vi "Plot Update Cursor 3D Surface.vi"(8 "Cursor XYZ":T1, 11 "3D Surface":refnum<vi>) -> ()   [LabVIEW 2016]
uses:
  <vilib>/Math Plots/3D Math Plots/3D Surface/3D Surface XCtrl/3D Surface.xctl
  <vilib>/addons/Software Calibration Management/xSCM/Controls/TLU2D.ctl
  <vilib>/Math Plots/3D Math Plots/3D Plot/3D Plot/Typedef/Sprite Type.ctl
  <vilib>/Math Plots/3D Math Plots/3D Plot/3D Plot/3D Plot.lvclass
  <vilib>/addons/Software Calibration Management/xSCM/SCM-API.lvlib
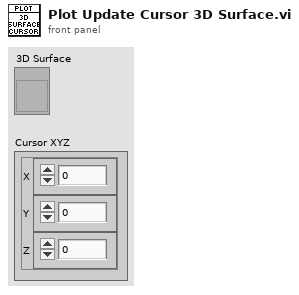
[diagram p1: front panel]
types:
  T1 = typedef "SCM-API.lvlib/TLU2D.ctl" = cluster{"X":sgl, "Y":sgl, "Z":sgl}
  T2 = typedef "3D Plot.lvclass/Sprite Type.ctl" = enum16{"None", "Empty Square", "Solid Square", "Empty Diamond", "Solid Diamond", "Empty Circle", "Solid Circle", "Asterisk", "Bold X", "Wireframe Sphere", "Solid Sphere", "Wireframe Cube", "Solid Cube"}
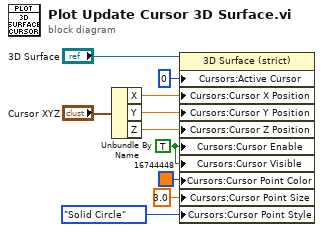
[diagram p0: block diagram]
diagram:
  w4 = TRUE ("Cursors:General:Cursor Enable")
  n1 = Unbundle By Name("Cursor XYZ") -> ("X"=w8:sgl, "Y"=w7:sgl, "Z"=w6:sgl)
  n2 = property class="3D Surface (strict)"(reference="3D Surface", "Cursors:Active Cursor"=0, "Cursors:Cursor X Position"=w8, "Cursors:Cursor Y Position"=w7, "Cursors:Cursor Z Position"=w6, "Cursors:Cursor Enable"=w4, "Cursors:Cursor Visible"=w4, "Cursors:Cursor Point Color"=u32 16744448 ("Cursors:Point:Cursor Point Color"), "Cursors:Cursor Point Size"=sgl 3.0 ("Cursors:Point:Cursor Point Size"), "Cursors:Cursor Point Style"=Sprite_Type."Solid Circle" ("Cursors:Point:Cursor Point Style")) -> ()  [unwired: 1 in, 2 out]
